vi "NMEA Example - data.vi"() -> ()   [LabVIEW 2019]
uses:
  NMEA_GPVTG-data.ctl
  NMEA_Mode.ctl
  NMEA_GPRMC-data.ctl
  NMEA_LatitudeDirection.ctl
  NMEA_LongitudeDirection.ctl
  NMEA_GPGGA-data.ctl
  NMEA_GPS-Quality.ctl
  NMEA.lvlib
panel:
  in  "test string":string
  in  "data":bool
  in  "Samples":string="$GPRMC,015848.1,A,3717.48964,N,12708.88920,E,000.11,001.6,030320,008.5,W,A*2C\n$GPGGA,015848.1,3717.48964,N,12708.88920,E,1,07,1.5,162.8,M,22.2,M,,*53\n$GPVTG,001.6,T,010.1,M,000.11,N,0000.20,K,A*16\n$GPRMC,015848.2,A,3717.48964,N,12708.88920,E,000.10,001.6,030320,008.5,W,A*2E\n$GPGGA,015848.2,3717.48964,N,12708.88920,E,1,07,1.5,162.8,M,22.2,M,,*50\n$GPVTG,001.6,T,010.1,M,000.10,N,0000.18,K,A*1C\n$GPRMC,015848.3,A,3717.48964,N,12708.88920,E,000.10,001.6,030320,008.5,W,A*2F\n$GPGGA,015848.3,3717.48964,N,12708.88920,E,1,07,1.5,162.8,M,22.2,M,,*51\n$GPVTG,001.6,T,010.1,M,000.10,N,0000.19,K,A*1D\n$GPRMC,015848.4,A,3717.48964,N,12708.88920,E,000.10,001.6,030320,008.5,W,A*28\n$GPGGA,015848.4,3717.48964,N,12708.88920,E,1,07,1.5,162.8,M,22.2,M,,*56\n$GPVTG,001.6,T,010.1,M,000.10,N,0000.18,K,A*1C\n$GPRMC,015848.5,A,3717.48964,N,12708.88920,E,000.10,001.6,030320,008.5,W,A*29\n$GPGGA,015848.5,3717.48964,N,12708.88920,E,1,06,1.8,162.8,M,22.2,M,,*5B\n$GPVTG,001.6,T,010.1,M,000.10,N,0000.18,K,A*1C\n$GPRMC,015848.6,A,3717.48964,N,12708.88920,E,000.09,001.6,030320,008.5,W,A*22\n$GPGGA,015848.6,3717.48964,N,12708.88920,E,1,06,1.8,162.8,M,22.2,M,,*58\n$GPVTG,001.6,T,010.1,M,000.09,N,0000.17,K,A*1B\n$GPRMC,015848.7,A,3717.48968,N,12708.88918,E,000.09,001.6,030320,008.5,W,A*24\n$GPGGA,015848.7,3717.48968,N,12708.88918,E,1,08,1.0,162.8,M,22.2,M,,*58\n$GPVTG,001.6,T,010.1,M,000.09,N,0000.17,K,A*1B\n$GPRMC,015848.8,A,3717.48968,N,12708.88918,E,000.09,001.6,030320,008.5,W,A*2B\n$GPGGA,015848.8,3717.48968,N,12708.88918,E,1,08,1.0,162.8,M,22.2,M,,*57\n$GPVTG,001.6,T,010.1,M,000.09,N,0000.17,K,A*1B\n$GPRMC,015848.9,A,3717.48968,N,12708.88918,E,000.10,001.6,030320,008.5,W,A*22\n$GPGGA,015848.9,3717.48968,N,12708.88918,E,1,08,1.0,162.8,M,22.2,M,,*56\n$GPVTG,001.6,T,010.1,M,000.10,N,0000.19,K,A*1D\n$GPRMC,015849.0,A,3717.48968,N,12708.88918,E,000.12,001.6,030320,008.5,W,A*28\n$GPGGA,015849.0,3717.48968,N,12708.88918,E,1,07,1.0,162.8,M,22.2,M,,*51\n$GPVTG,001.6,T,010.1,M,000.12,N,0000.22,K,A*17\n$GPGSA,A,3,25,22,31,12,32,20,10,,,,,,1.7,1.0,1.4*34\n$GPGSV,2,1,07,25,63,060,32,22,15,315,38,31,43,281,42,12,27,043,22*79\n$GPGSV,2,2,07,32,83,025,31,20,06,176,25,10,31,195,19*44\n$GPRMC,015849.1,A,3717.48968,N,12708.88918,E,000.12,001.6,030320,008.5,W,A*29"
  in  "Data file path":path
  out "$GPGGA-message_OUT":T1={"TimeStamp"=timestamp(0 s since 1904-01-01), "Latitude"=0.0, "Latitude-Direction"=enum."", "Longitude"=1.0, "Longitude-Direction"=enum."", "GPS-Quality"=enum."GPS fix (SPS)", "Number of Satellites"=0, "Horizontal Dilution of Precision"=0.0, "Altitude above Mean-Sea-Level"=0.0, "Geoidal separation"=0.0, "Time since last DGPS update"=0.0, "DGPS reference station ID"=0} {"Time since last DGPS update" format="%.02f [s]"; "Geoidal separation" format="%.02f [m]"; "Altitude above Mean-Sea-Level" format="%.02f [m]"; "Horizontal Dilution of Precision" format="%.02f [HDOP]"; "Longitude" format="%0.4f [long]"; "Latitude" format="%.04f [lat]"; "TimeStamp" format="%<%.2X>T"}
  out "TX LAT":dbl
  out "TX LONG":dbl
  out "Data":string[][](table)
  out "$GPRMC-message_OUT":T5={"TimeStamp"=timestamp(0 s since 1904-01-01), "Validity"=FALSE, "Latitude"=0.0, "Latitude-Direction"=enum."North", "Longitude"=0.0, "Longitude-Direction"=enum."East", "Speed in knots"=0.0, "True course"=0.0, "Date Stamp"=timestamp(0 s since 1904-01-01), "Magnetic Variation (East/West)"=0.0} {"Magnetic Variation (East/West)" format="%.02f [deg]"; "Date Stamp" format="%<%x>T"; "True course" format="%.02f [deg]"; "Speed in knots" format="%.02f [kts]"; "Longitude" format="%0.4f [long]"; "Latitude" format="%.04f [lat]"; "TimeStamp" format="%<%.2X>T"}
  out "$GPVTG-message_OUT":T6={"True Course over Ground"=0.0, "Magnetic Course over Ground"=0.0, "Speed over Ground in knots"=0.0, "Speed over Ground in km/h"=1.0, "Mode"=""} {"Speed over Ground in km/h" format="%.02f [km/h]"; "Speed over Ground in knots" format="%.02f [kts]"; "Magnetic Course over Ground" format="%.02f [deg]"; "True Course over Ground" format="%.02f [deg]"}
  out "Raw data GPS":string
  in  "Stop":bool
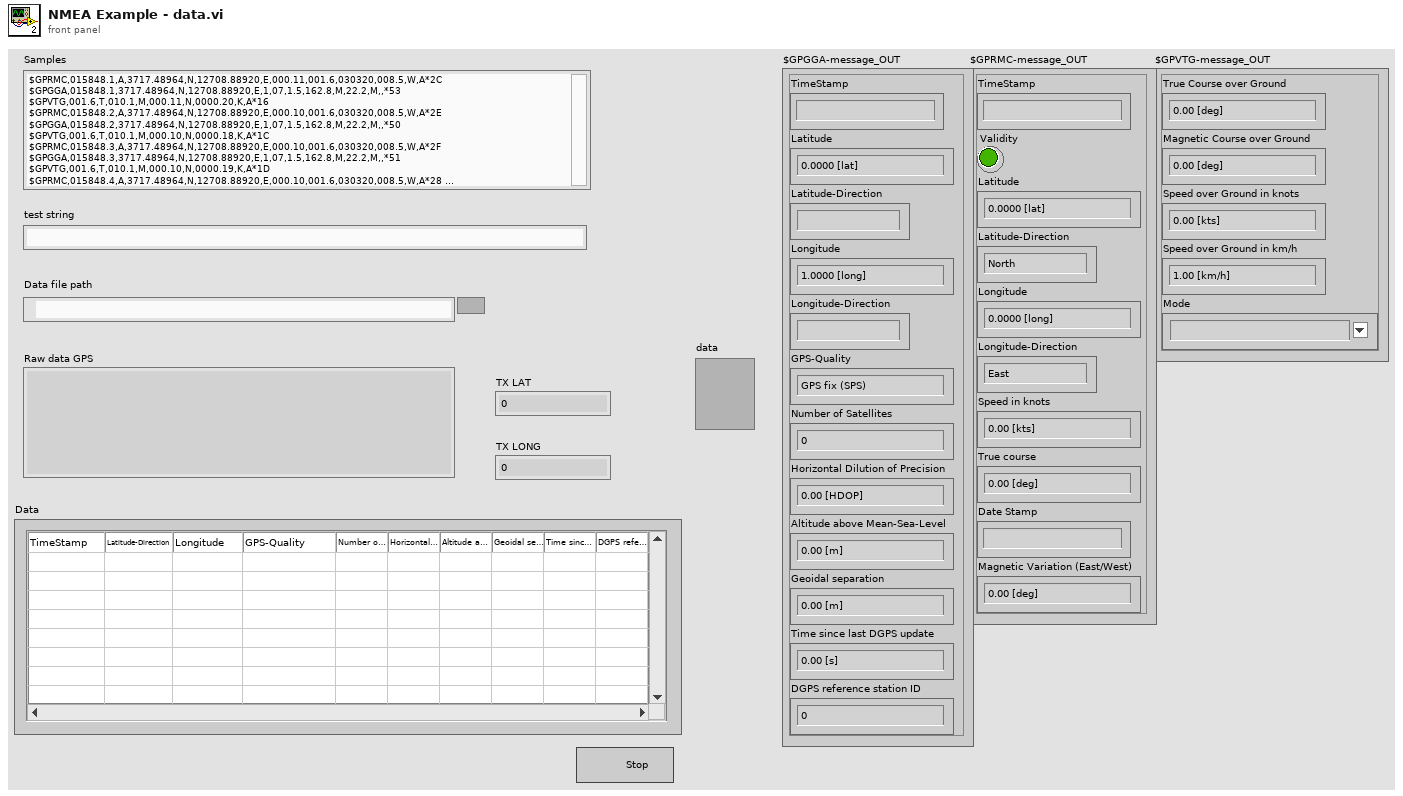
[diagram p1: front panel]
types:
  T1 = typedef "NMEA.lvlib/NMEA_GPGGA-data.ctl" = cluster{"TimeStamp":timestamp, "Latitude":dbl, "Latitude-Direction":T2, "Longitude":dbl, "Longitude-Direction":T3, "GPS-Quality":T4, "Number of Satellites":i32, "Horizontal Dilution of Precision":dbl, "Altitude above Mean-Sea-Level":dbl, "Geoidal separation":dbl, "Time since last DGPS update":dbl, "DGPS reference station ID":i32}
  T2 = typedef "NMEA.lvlib/NMEA_LatitudeDirection.ctl" = enum16{"", "North", "South"}
  T3 = typedef "NMEA.lvlib/NMEA_LongitudeDirection.ctl" = enum16{"", "East", "West"}
  T4 = typedef "NMEA.lvlib/NMEA_GPS-Quality.ctl" = enum16{"Invalid", "GPS fix (SPS)", "DGPS fix", "PPS fix", "Real Time Kinematic", "Float RTK", "estimated", "Manual input mode", "Simulation mode"}
  T5 = typedef "NMEA.lvlib/NMEA_GPRMC-data.ctl" = cluster{"TimeStamp":timestamp, "Validity":bool, "Latitude":dbl, "Latitude-Direction":T2, "Longitude":dbl, "Longitude-Direction":T3, "Speed in knots":dbl, "True course":dbl, "Date Stamp":timestamp, "Magnetic Variation (East/West)":dbl}
  T6 = typedef "NMEA.lvlib/NMEA_GPVTG-data.ctl" = cluster{"True Course over Ground":dbl, "Magnetic Course over Ground":dbl, "Speed over Ground in knots":dbl, "Speed over Ground in km/h":dbl, "Mode":T7}
  T7 = typedef "NMEA.lvlib/NMEA_Mode.ctl" = string
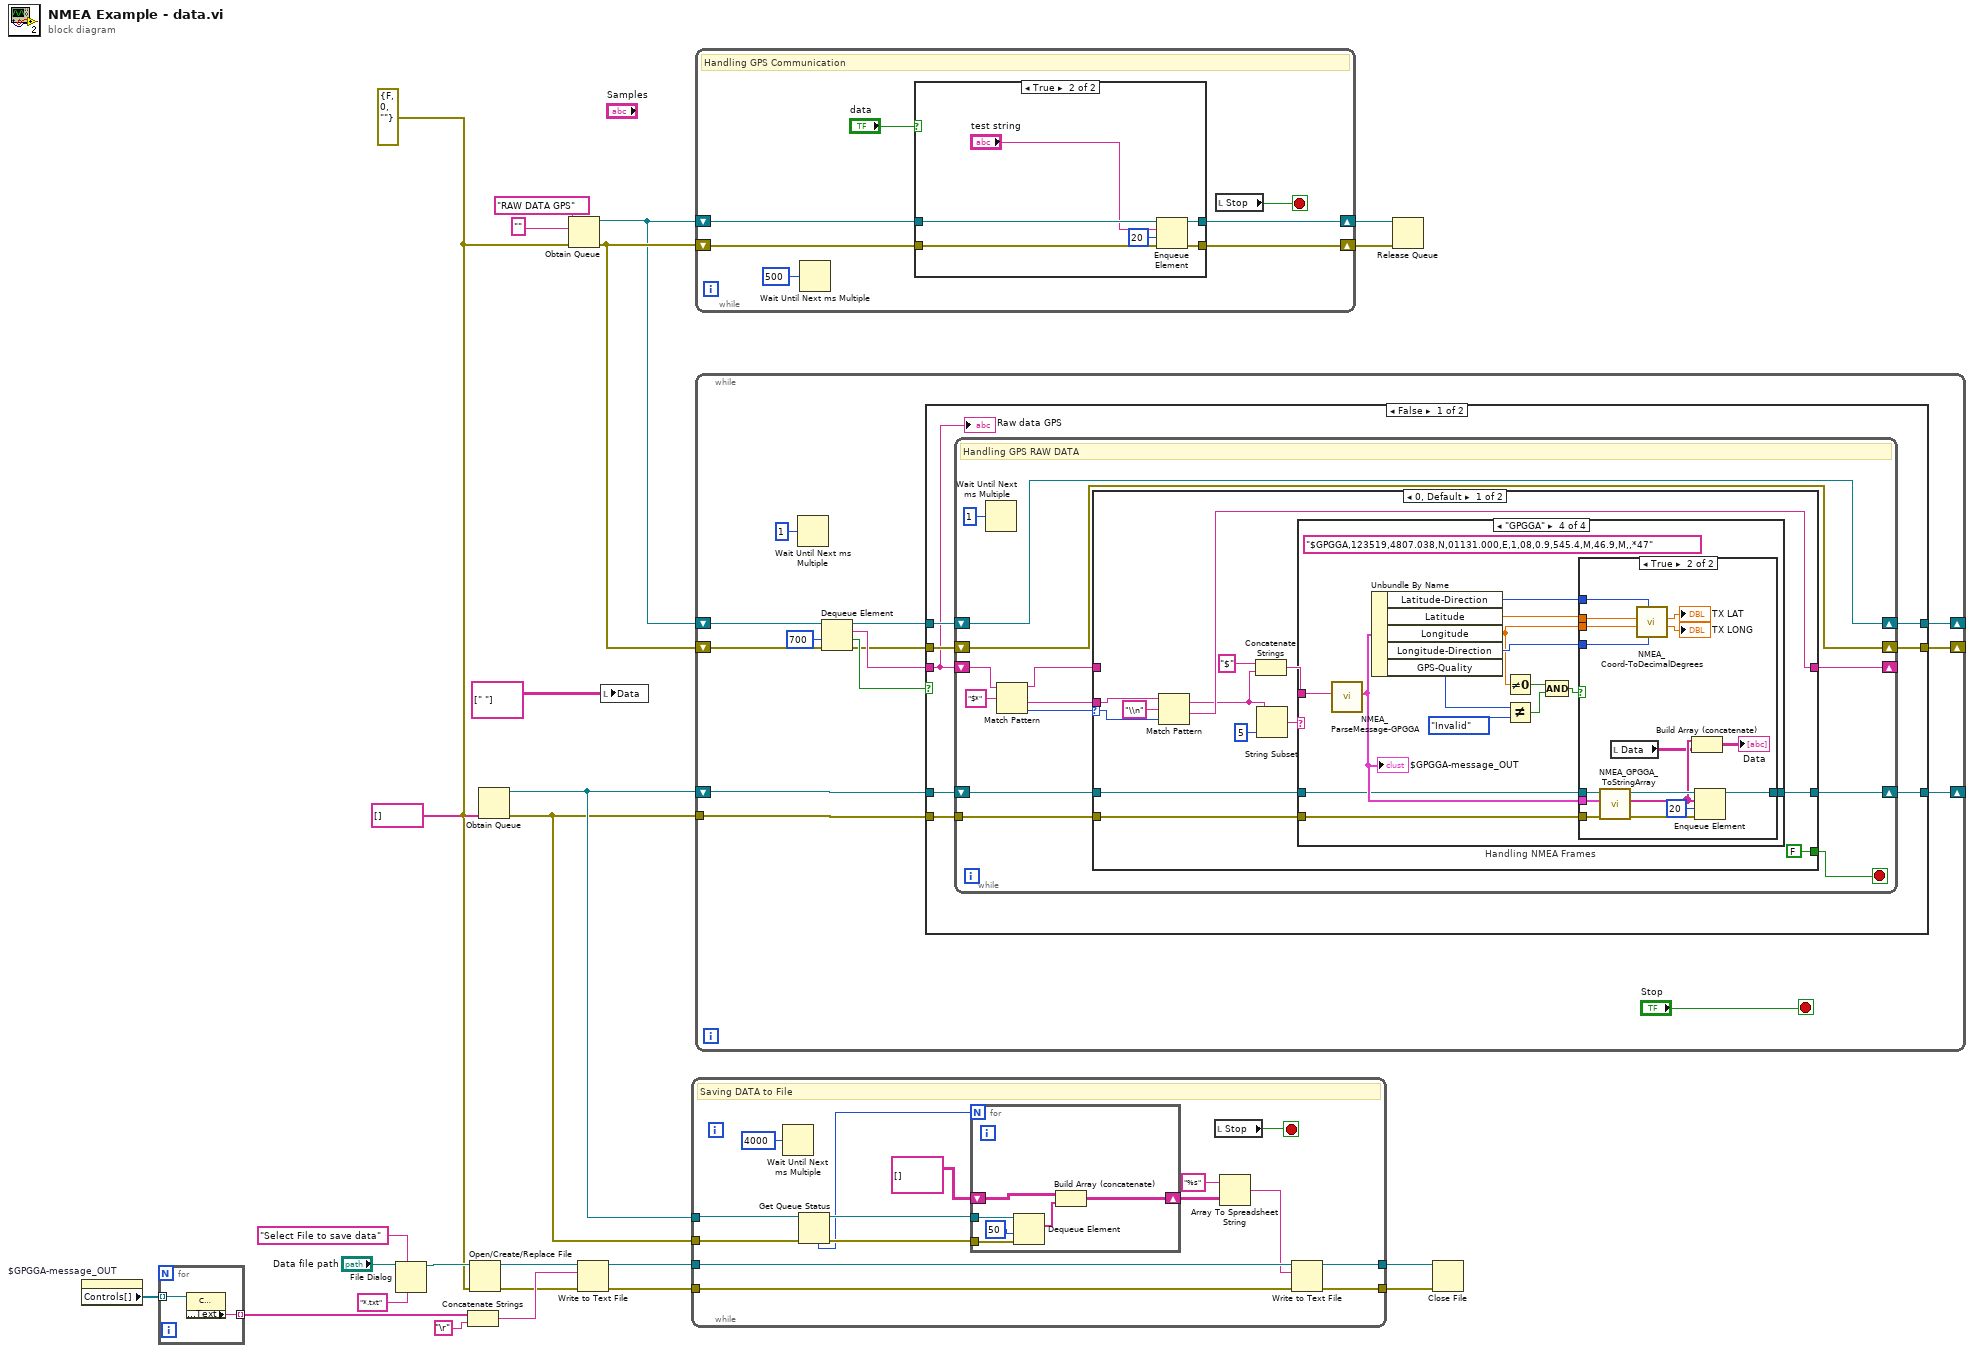
[diagram p0: block diagram]
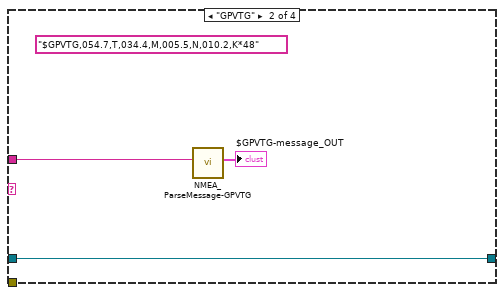
[diagram p4: hidden frame]
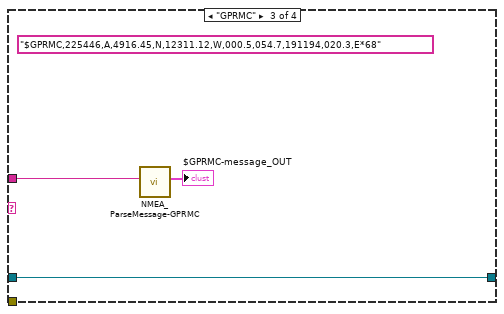
[diagram p5: hidden frame]
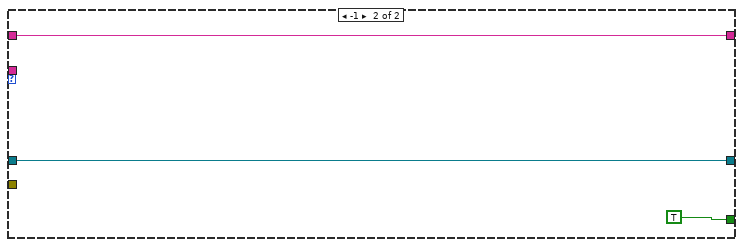
[diagram p7: hidden frame]
diagram:
  w1 = errorcluster {"status"=FALSE, "code"=0, "source"=""} ("error constant")
  n1 = property on="$GPGGA-message_OUT" class="Clust (strict)"() -> ("Controls[]"=w10:refnum<vi>[])  [unwired: 2 in, 2 out]
  n2 = for {
    tunnel: w10 -> [w27] mode=indexing
    tunnel: [w26] -> w7 mode=indexing
    n3 = property class="Cmde"(reference=w27) -> ("Label.Text"=w26:string)  [unwired: 1 in, 2 out]
  }
  n4 = File Dialog(6:"*.txt" ("filtre (tous les fichiers)"), 7:"Select File to save data" ("message"), 11:"Data file path") -> (3:w4:path)  [unwired: 4 in, 3 out]
  n5 = Concatenate Strings(w7, "\r") -> (w22:string)
  n6 = Open/Create/Replace File(file path (use dialog)=w4, error in=w1) -> (refnum out=w13:refnum<file>, error out=w12:errorcluster)  [unwired: 4 in, 1 out]
  n7 = Obtain Queue(element data type=string[] [], error in (no error)=w1) -> (queue out=w21:refnum<queue>, error out=w20:errorcluster)  [unwired: 3 in, 1 out]
  n8 = Obtain Queue(name (unnamed)="RAW DATA GPS" ("nom (aucun)"), element data type="" ("expression régulière"), error in (no error)=w1) -> (queue out=w16:refnum<queue>, error out=w25:errorcluster)  [unwired: 2 in, 1 out]
  n9 = Write to Text File(file (use dialog)=w13, text=w22, error in=w12) -> (refnum out=w23:refnum<file>, error out=w24:errorcluster)  [unwired: 1 in, 1 out]
  n10 = local write "Data"(string[][] [[" "]]) -> ()
  n11 = while {
    tunnel: [w42] -> w15
    tunnel: [w41] -> w14
    tunnel: w24 -> [w40]
    tunnel: w23 -> [w39]
    tunnel: w21 -> [w33]
    tunnel: w20 -> [w31]
    stop <- w28 stop-if-true
    # "Saving DATA to File"
    n12 = Wait Until Next ms Multiple(millisecond multiple=u32 4000 ("n millisecondes")) -> ()  [unwired: 1 out]
    n13 = Get Queue Status(queue=w33, error in (no error)=w31) -> (queue out=w32:refnum<queue>, error out=w30:errorcluster, # elements in queue=w29:i32)  [unwired: 1 in, 5 out]
    n14 = for {
      N: w29 -> [_]
      shift-right: [w44] -> w37
      shift-left: string[][] [] -> [w48]
      tunnel: w32 -> [w47]
      tunnel: w30 -> [w46]
      n15 = Dequeue Element(queue=w47, timeout in ms (-1)=50 ("timeout en ms (-1)"), error in (no error)=w46) -> (element=w45:string[])  [unwired: 3 out]
      n16 = Build Array (concatenate)(w48, w45) -> (w44:string[][])
    }
    n17 = local read "Stop"() -> (w28:bool)
    n18 = Array To Spreadsheet String(array=w37, 3:"%s" ("format string")) -> (spreadsheet string=w36:string)  [unwired: 1 in]
    n19 = Write to Text File(file (use dialog)=w39, text=w36, error in=w40) -> (refnum out=w42:refnum<file>, error out=w41:errorcluster)  [unwired: 1 in, 1 out]
  }
  n20 = while {
    shift-right: [w52] -> w18
    shift-left: w25 -> [w54]
    shift-right: [w53] -> w17
    shift-left: w16 -> [w55]
    stop <- w50 stop-if-true
    # "Handling GPS Communication"
    n21 = Wait Until Next ms Multiple(millisecond multiple=u32 500 ("attente (ms)")) -> ()  [unwired: 1 out]
    n22 = case shown="True" "data" {
      tunnel: w55 -> [w56 w63]
      tunnel: w54 -> [w57 w62]
      tunnel: [w56 w61] -> w53
      tunnel: [w57 w60] -> w52
      frame False {
      }
      frame True {
        n23 = Enqueue Element(queue=w63, element="test string", timeout in ms (-1)=20 ("timeout en ms (-1)"), error in (no error)=w62) -> (queue out=w61:refnum<queue>, error out=w60:errorcluster)  [unwired: 1 out]
      }
    }
    n24 = local read "Stop"() -> (w50:bool)
  }
  n25 = while {
    tunnel: w20 -> [w73]
    shift-right: [w71] -> _
    shift-left: w16 -> [w72]
    shift-right: [w67] -> _
    shift-left: w21 -> [w74]
    shift-right: [w66] -> _
    shift-left: w25 -> [w77]
    stop <- "Stop" stop-if-true
    n26 = Wait Until Next ms Multiple(millisecond multiple=u32 1 ("n millisecondes")) -> ()  [unwired: 1 out]
    n27 = Dequeue Element(queue=w72, timeout in ms (-1)=700 ("timeout en ms (-1)"), error in (no error)=w77) -> (queue out=w70:refnum<queue>, element=w76:string, timed out?=w68:bool, error out=w65:errorcluster)
    n28 = case shown="False" w68 {
      tunnel: w76 -> [w78 _]
      tunnel: w74 -> [w85 w152]
      tunnel: w73 -> [w84 _]
      tunnel: [w83 w153] -> w71
      tunnel: w70 -> [w82 w153]
      tunnel: [w81 w152] -> w67
      tunnel: [w80 w151] -> w66
      tunnel: w65 -> [w79 w151]
      frame False {
        n29 = while {
          shift-right: [w96] -> _
          shift-left: w78 -> [w87]
          tunnel: w84 -> [w92]
          shift-right: [w91] -> w83
          shift-left: w82 -> [w91]
          shift-right: [w89] -> w81
          shift-left: w85 -> [w93]
          shift-right: [w88] -> w80
          shift-left: w79 -> [w88]
          stop <- w90 stop-if-true
          # "Handling GPS RAW DATA"
          n30 = Wait Until Next ms Multiple(millisecond multiple=u32 1 ("n millisecondes")) -> ()  [unwired: 1 out]
          n31 = Match Pattern(string=w87, regular expression="$*" ("expression régulière")) -> (before substring=w86:string, after substring=w95:string, offset past match=w97:i32)  [unwired: 1 in, 1 out]
          n32 = case shown="0, Default" w97 {
            selector: w97 -> [w108 _]
            tunnel: [w107 w148] -> w96
            tunnel: w95 -> [w109 _]
            tunnel: [FALSE TRUE] -> w90
            tunnel: w93 -> [w102 w149]
            tunnel: w92 -> [w101 _]
            tunnel: [w99 w149] -> w89
            tunnel: w86 -> [_ w148]
            frame 0, Default {
              n33 = Match Pattern(string=w109, regular expression="\\n" ("expression régulière"), offset (0)=w108) -> (before substring=w106:string, after substring=w107:string)  [unwired: 2 out]
              n34 = Concatenate Strings("$" ("expression régulière"), w106) -> (w104:string)
              n35 = String Subset(string=w106, length (rest)=5 ("longueur (reste)")) -> (substring=w110:string)  [unwired: 1 in]
              n36 = case "Handling NMEA Frames" shown="\"GPGGA\"" w110 {
                tunnel: w104 -> [_ w114 w117 w132]
                tunnel: w102 -> [w112 w113 w116 w127]
                tunnel: w101 -> [_ _ _ w126]
                tunnel: [w112 w113 w116 w125] -> w99
                frame " ", Default {
                }
                frame "GPVTG" {
                  (unwired) "$GPVTG,054.7,T,034.4,M,005.5,N,010.2,K*48" ("$GPVTG-message_IN")
                  n37 = call "NMEA_ParseMessage-GPVTG.vi"("$GPVTG-message_IN"=w114) -> ("$GPVTG-message_OUT"=→"$GPVTG-message_OUT":T6)  [unwired: 9 in, 1 out]
                }
                frame "GPRMC" {
                  (unwired) "$GPRMC,225446,A,4916.45,N,12311.12,W,000.5,054.7,191194,020.3,E*68" ("$GPRMC-message_IN")
                  n38 = call "NMEA_ParseMessage-GPRMC.vi"("$GPRMC-message_IN"=w117) -> ("$GPRMC-message_OUT"=→"$GPRMC-message_OUT":T5)  [unwired: 9 in, 1 out]
                }
                frame "GPGGA" {
                  (unwired) "$GPGGA,123519,4807.038,N,01131.000,E,1,08,0.9,545.4,M,46.9,M,,*47" ("data out")
                  n39 = call "NMEA_ParseMessage-GPGGA.vi"("$GPGGA-message_IN"=w132) -> ("$GPGGA-message_OUT"=w128:T1)  [unwired: 9 in, 1 out]
                  "$GPGGA-message_OUT" <- w128
                  n40 = Unbundle By Name(w128) -> ("Latitude-Direction"=w129:T2, "Latitude"=w130:dbl, "Longitude"=w124:dbl, "Longitude-Direction"=w131:T3, "GPS-Quality"=w119:T4)
                  n41 = Not Equal To 0?(x=w124) -> (x != 0?=w122:bool)
                  n42 = Not Equal?(x=w119, y=NMEA_GPS-Quality."Invalid" ("GPS-Quality")) -> (x != y?=w120:bool)
                  n43 = Compound Arithmetic op=AND(w122, w120) -> (w123:bool)
                  n44 = case shown="True" w123 {
                    tunnel: w131 -> [_ w145]
                    tunnel: w130 -> [_ w135]
                    tunnel: w129 -> [_ w134]
                    tunnel: w128 -> [_ w144]
                    tunnel: w127 -> [w133 w143]
                    tunnel: w126 -> [_ w142]
                    tunnel: [w133 w138] -> w125
                    tunnel: w124 -> [_ w136]
                    frame False {
                    }
                    frame True {
                      n45 = call "NMEA_GPGGA_ToStringArray.vi"("$GPGGA-message_IN"=w144) -> ("$GPGGA-message_OUT"=w140:string[])  [unwired: 9 in, 1 out]
                      n46 = local read "Data"() -> (w139:string[][])
                      n47 = call "NMEA_Coord-ToDecimalDegrees.vi"("Longitude-Direction"=w145, "Latitude-Direction"=w134, "Longitude"=w136, "Latitude"=w135) -> ("Longitude"=→"TX LONG":dbl, "Latitude"=→"TX LAT":dbl)  [unwired: 6 in]
                      n48 = Build Array (concatenate)(w140, w139) -> (→"Data":string[][])
                      n49 = Enqueue Element(queue=w143, element=w140, timeout in ms (-1)=20 ("timeout en ms (-1)"), error in (no error)=w142) -> (queue out=w138:refnum<queue>)  [unwired: 2 out]
                    }
                  }
                }
              }
            }
            frame -1 {
            }
          }
        }
        "Raw data GPS" <- w78
      }
      frame True {
      }
    }
  }
  n50 = Release Queue(queue=w17, error in (no error)=w18) -> ()  [unwired: 1 in, 3 out]
  n51 = Close File(refnum=w15, error in=w14) -> ()  [unwired: 2 out]
